vi "initialize manifold config array control (sub-vi).vi"(8 "error in (no error)":errorcluster, 9 "ports per stimulator (8)":i32=8, 10 "num stimulators (3)":i32=3, 11 "stimulator config array refnum":refnum<vi>) -> (0 "error out":errorcluster, 3 "stimulator config array refnum out":refnum<vi>)   [LabVIEW 2021]
uses:
  type-defs/manifold configuration cluster (type def).ctl
  type-defs/manifold selection.ctl
  type-defs/single port single odor cluster.ctl
  type-defs/port number (type def).ctl
  type-defs/odor selection (type def).ctl
  type-defs/odor color (type def).ctl
  type-defs/odor color enum (type def).ctl
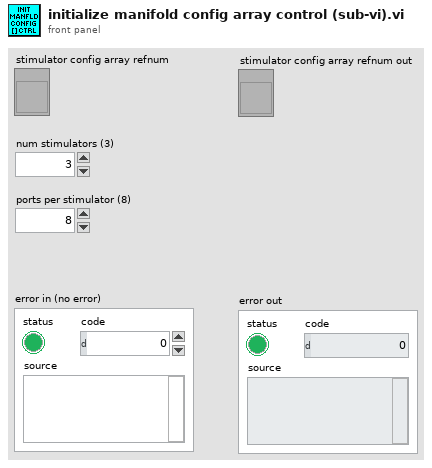
[diagram p1: front panel]
types:
  T1 = typedef "manifold configuration cluster (type def).ctl" = cluster{"position:":T2, "port connections:":T3[]}
  T2 = typedef "manifold selection.ctl" = enum16{"left", "middle", "right"}
  T3 = typedef "single port single odor cluster.ctl" = cluster{"port number":T4, "connected odor":T5, "error":bool, "odor color":T6}
  T4 = typedef "port number (type def).ctl" = enum16{"port 1", "port 2", "port 3", "port 4", "port 5", "port 6", "port 7", "port 8"}
  T5 = typedef "odor selection (type def).ctl" = enum16{"[none]", "odor 1", "odor 2", "odor 3", "odor 4", "odor 5", "odor 6", "odor 7", "odor 8", "odor 9", "odor 10"}
  T6 = typedef "odor color (type def).ctl" = u16
  T7 = typedef "odor color enum (type def).ctl" = enum16{"white", "blue", "red", "orange", "yellow", "green", "magenta", "brown", "black", "[none]"}
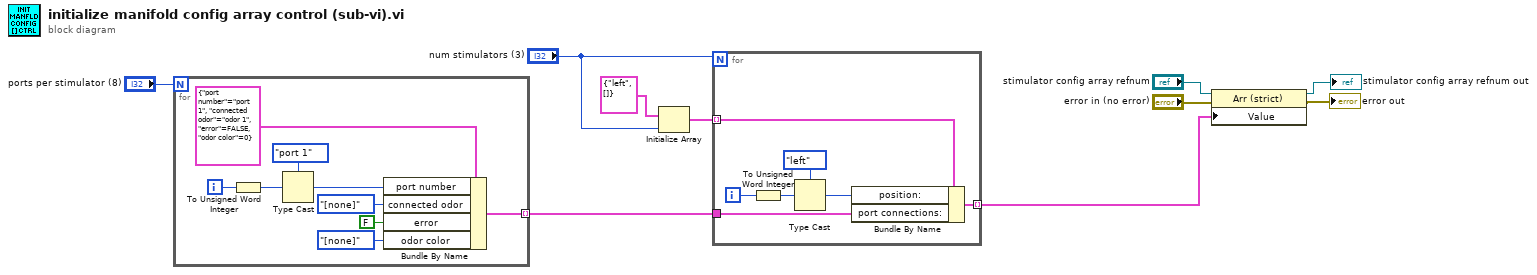
[diagram p0: block diagram]
diagram:
  n1 = for {
    N: "ports per stimulator (8)" -> [_]
    tunnel: [w12] -> w6 mode=indexing
    i -> [w15]
    n2 = To Unsigned Word Integer(number=w15) -> (unsigned 16bit integer=w11:u16)
    n3 = Type Cast(type=port_number_(type_def)."port 1" ("port number"), x=w11) -> (*(type *) &x=w14:T4)
    n4 = Bundle By Name(cluster=T3 {"port number"=enum."port 1", "connected odor"=enum."odor 1", "error"=FALSE, "odor color"=0} ("port-odor cluster"), "port number"=w14, "connected odor"=odor_selection_(type_def)."[none]", "error"=FALSE, "odor color"=odor_color_enum_(type_def)."[none]" ("Enum")) -> (w12:T3)
  }
  n5 = Initialize Array(T1 {"position:"=enum."left", "port connections:"=[]} ("stimulator configuration cluster"), "num stimulators (3)") -> (w8:T1[])
  n6 = for {
    N: "num stimulators (3)" -> [_]
    tunnel: w8 -> [w26] mode=indexing
    tunnel: w6 -> [w22]
    tunnel: [w21] -> w3 mode=indexing
    i -> [w24]
    n7 = To Unsigned Word Integer(number=w24) -> (unsigned 16bit integer=w20:u16)
    n8 = Type Cast(type=manifold_selection."left" ("position:"), x=w20) -> (*(type *) &x=w23:T2)
    n9 = Bundle By Name(cluster=w26, "position:"=w23, "port connections:"=w22) -> (w21:T1)
  }
  n10 = property class="Arr (strict)"(reference="stimulator config array refnum", error in="error in (no error)", "Value"=w3) -> (reference out=→"stimulator config array refnum out":refnum<vi>, error out=→"error out":errorcluster)
